vi "Set scope v0.2.vi"(2 "error in (no error)":errorcluster, 3 "input commands":string=":WGEN:frequency 5.000000E+2\n:WGEN:VOLTage 5E+0\n :WGEN:OUTPut 1\n:WGEN:VOLTage:OFFSet 1e-6\n:WGEN:OUTPut:LOAD ONEMeg\n:wgen:function sinusoid\n:WGEN:OUTPut:POLarity 0\n:AUToscale\n:channel1:bwlimit 0\n:channel1:coupling AC\n:channel1:display 1\n:channel1:invert 0\n:channel1:offset 0\n:channel2:bwlimit 0\n:channel2:coupling AC\n:channel2:display 1\n:channel2:invert 0\n:channel2:offset 0", 4 "VISA resource name in":refnum<visa-resource-name>="USB0::0x2A8D::0x1797::CN58056431::0::INSTR") -> (0 "error out":errorcluster={"status"=TRUE, "code"=-1073807247, "source"="VISA Write in Set scope.vi->Frequency sweep (simple).vi"}, 1 "VISA resource name out":refnum<visa-resource-name>="USB0::0x2A8D::0x1797::CN58056431::0::INSTR")   [LabVIEW 2017]
panel:
  out "parsed commands":string[](array[string])
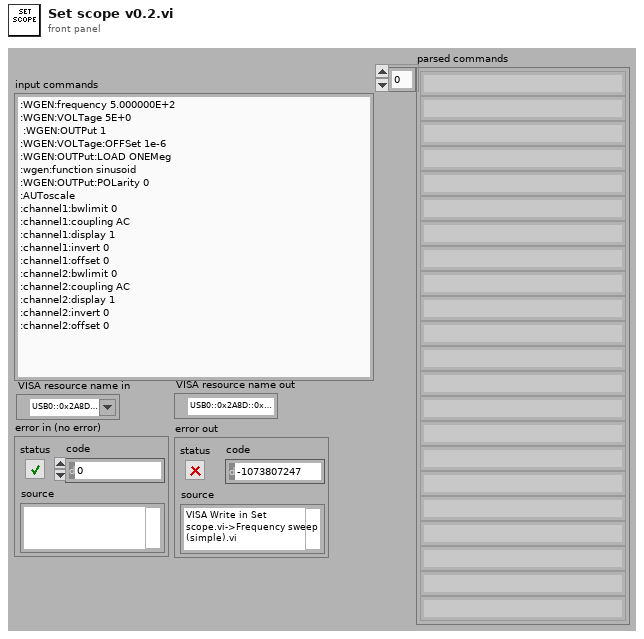
[diagram p1: front panel]
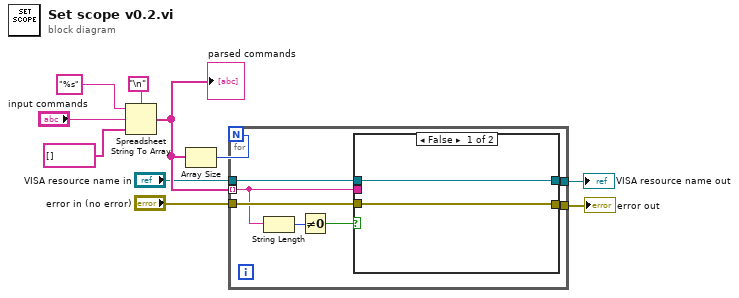
[diagram p0: block diagram]
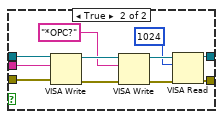
[diagram p2: hidden frame]
diagram:
  n1 = Spreadsheet String To Array(delimiter (Tab)="\n", format string="%s", spreadsheet string="input commands", array type (2D Dbl)=string[] []) -> (array=w5:string[])
  "parsed commands" <- w5
  n2 = Array Size(array=w5) -> (size(s)=w6:i32)
  n3 = for {
    N: w6 -> [_]
    tunnel: w5 -> [w13] mode=indexing
    tunnel: "VISA resource name in" -> [w17]
    tunnel: "error in (no error)" -> [w16]
    tunnel: [w15] -> w2
    tunnel: [w14] -> w1
    n4 = String Length(string=w13) -> (length=w12:i32)
    n5 = Not Equal To 0?(x=w12) -> (x != 0?=w11:bool)
    n6 = case shown="False" w11 {
      tunnel: w17 -> [w19 w30]
      tunnel: w16 -> [w18 w29]
      tunnel: [w19 w22] -> w15
      tunnel: [w18 w21] -> w14
      tunnel: w13 -> [_ w20]
      frame False {
      }
      frame True {
        n7 = VISA Write(VISA resource name=w30, write buffer=w20, error in (no error)=w29) -> (VISA resource name out=w27:refnum<visa-resource-name>, error out=w28:errorcluster)  [unwired: 1 out]
        n8 = VISA Write(VISA resource name=w27, write buffer="*OPC?", error in (no error)=w28) -> (VISA resource name out=w24:refnum<visa-resource-name>, error out=w25:errorcluster)  [unwired: 1 out]
        n9 = VISA Read(VISA resource name=w24, byte count=u32 1024, error in (no error)=w25) -> (VISA resource name out=w22:refnum<visa-resource-name>, error out=w21:errorcluster)  [unwired: 2 out]
      }
    }
  }
  "VISA resource name out" <- w2
  "error out" <- w1
